vi "Not A Gate.vi"(1 "gate":T1) -> (0 "nor a gate?":bool)   [LabVIEW 2015, in "Gates.lvlib"]
doc: "Returns TRUE if <B>gate</B> is not a valid gate refnum."
uses:
  Gates.lvlib
  Gate.ctl
  Gate Pass.ctl
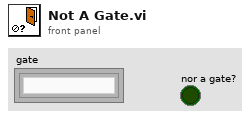
[diagram p1: front panel]
types:
  T1 = typedef "Gates.lvlib/Gate.ctl" = refnum<k1>
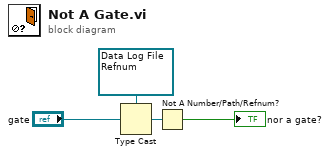
[diagram p0: block diagram]
diagram:
  w4 = refnum<queue> refnum items=["Gate Pass"] ("queue out")
  n1 = Type Cast(type=w4, x="gate") -> (*(type *) &x=w2:refnum<queue>)
  n2 = Not A Number/Path/Refnum?(number/path/refnum=w2) -> (NaN/Path/Refnum?=→"nor a gate?":bool)
